vi "Configurate Channel Osciloscope.vi"(8 "error in (no error)":errorcluster, 10 "Configurate Channel--cluster":T1={"Tektronix"={"Enable Channel (True)"=TRUE, "Channel (0: Channel 1)"=0, "Vertical Coupling (1: DC)"=1, "Probe Attenuation (10: 10X)"=10, "Vertical Range (10.0 V/div)"=10.0, "Vertical Offset (0.0 divs)"=0.0, "Bandwidth (0: MAX Bandwidth)"=0}, "EDU-X-1002A"={"Vertical Scale (5.0 V)"=5.0, "Impedance (0: 1 MOhm)"=0, "Channel Name (0: Channel 1)"=0, "Coupling (1: DC)"=1, "Vertical Range (40.0 V)"=40.0, "Vertical Offset (0.0)"=0.0, "Probe Attenuation (1.0)"=1.0, "Vertical Setting (1: Vertical Range)"=1}} {"EDU-X-1002A"."Vertical Setting (1: Vertical Range)" items=["Vertical Scale", "Vertical Range"]; "EDU-X-1002A"."Coupling (1: DC)" items=["AC", "DC"]; "EDU-X-1002A"."Channel Name (0: Channel 1)" items=["Channel 1", "Channel 2", "Channel 3", "Channel 4"]; "EDU-X-1002A"."Impedance (0: 1 MOhm)" items=["1 MOhm", "50 Ohm"]; "Tektronix"."Bandwidth (0: MAX Bandwidth)" items=["MAX Bandwidth", "Unlimited"]; "Tektronix"."Probe Attenuation (10: 10X)" items=["1"=1, "10"=10, "20"=20, "50"=50, "100"=100, "500"=500, "1000"=1000]; "Tektronix"."Vertical Coupling (1: DC)" items=["AC", "DC", "Ground"]; "Tektronix"."Channel (0: Channel 1)" items=["Channel 1", "Channel 2", "Channel 3", "Channel 4", "Math", "Reference A", "Reference B", "Reference C", "Reference D"]}, 11 "EDU-X 1002A in":refnum<class "EDU-X 1002A.lvclass">) -> (0 "error out":errorcluster, 3 "EDU-X 1002A out":refnum<class "EDU-X 1002A.lvclass">)   [LabVIEW 2020, in "EDU-X 1002A.lvclass"]
uses:
  EDU-X 1002A.lvclass
  TypeDefs/ConfigurateCahnnel--cluster.ctl
  EDU-X 1002A.lvclass/EDU-X 1002A.ctl
  <instrlib>/Agilent 2000 3000 X-Series/Agilent 2000 3000 X-Series.lvlib
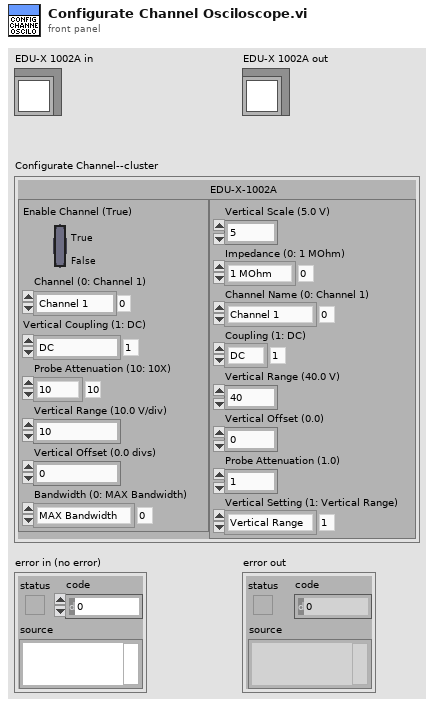
[diagram p1: front panel]
types:
  T1 = typedef "ConfigurateCahnnel--cluster.ctl" = cluster{"Tektronix":cluster{"Enable Channel (True)":bool, "Channel (0: Channel 1)":i32, "Vertical Coupling (1: DC)":i32, "Probe Attenuation (10: 10X)":i32, "Vertical Range (10.0 V/div)":dbl, "Vertical Offset (0.0 divs)":dbl, "Bandwidth (0: MAX Bandwidth)":i32}, "EDU-X-1002A":cluster{"Vertical Scale (5.0 V)":dbl, "Impedance (0: 1 MOhm)":i32, "Channel Name (0: Channel 1)":i32, "Coupling (1: DC)":i32, "Vertical Range (40.0 V)":dbl, "Vertical Offset (0.0)":dbl, "Probe Attenuation (1.0)":dbl, "Vertical Setting (1: Vertical Range)":i32}}
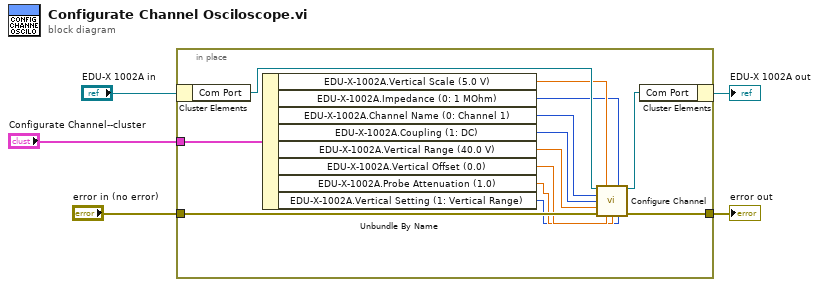
[diagram p0: block diagram]
diagram:
  n1 = in-place {
    in-place-border: [w16] -> w3
    in-place-border: "error in (no error)" -> [w15]
    in-place-border: "Configurate Channel--cluster" -> [w14]
    n2 = in-place-cluster #1("EDU-X 1002A in") -> ("Com Port"=w18:refnum<visa-resource-name>)
    n3 = Unbundle By Name(w14) -> ("EDU-X-1002A.Vertical Scale (5.0 V)"=w13:dbl, "EDU-X-1002A.Impedance (0: 1 MOhm)"=w12:i32, "EDU-X-1002A.Channel Name (0: Channel 1)"=w11:i32, "EDU-X-1002A.Coupling (1: DC)"=w10:i32, "EDU-X-1002A.Vertical Range (40.0 V)"=w9:dbl, "EDU-X-1002A.Vertical Offset (0.0)"=w8:dbl, "EDU-X-1002A.Probe Attenuation (1.0)"=w7:dbl, "EDU-X-1002A.Vertical Setting (1: Vertical Range)"=w6:i32)
    n4 = call <instrlib>:"Configure Channel.vi"("VISA resource name"=w18, "Vertical Scale (5.0 V)"=w13, "Impedance (0: 1 MOhm)"=w12, "Channel Name (0: Channel 1)"=w11, "Coupling (1: DC)"=w10, "Vertical Range (40.0 V)"=w9, "error in (no error)"=w15, "Vertical Offset (0.0)"=w8, "Probe Attenuation (1.0)"=w7, "Vertical Setting (1: Vertical Range)"=w6) -> ("VISA resource name out"=w17:refnum<visa-resource-name>, "error out"=w16:errorcluster)  [unwired: 4 in]
    n5 = in-place-cluster #1("Com Port"=w17) -> (→"EDU-X 1002A out":refnum<class "EDU-X 1002A.lvclass">)
  }
  "error out" <- w3
